vi "Handle.vi"(11 "Hello World Queue in":refnum<class "Hello World Queue.lvclass">) -> (2 "Destroy?":bool, 3 "Hello World Queue out":refnum<class "Hello World Queue.lvclass">)   [LabVIEW 2021, in "Hello World Queue.lvlib" / "Hello World Queue.lvclass"]
uses:
  Hello World Queue.lvclass
  Hello World Queue.lvclass/Hello World Queue.ctl
  jettl/Actor/Queue Actor/Queue Actor.lvclass
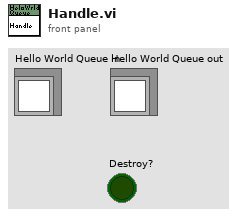
[diagram p1: front panel]
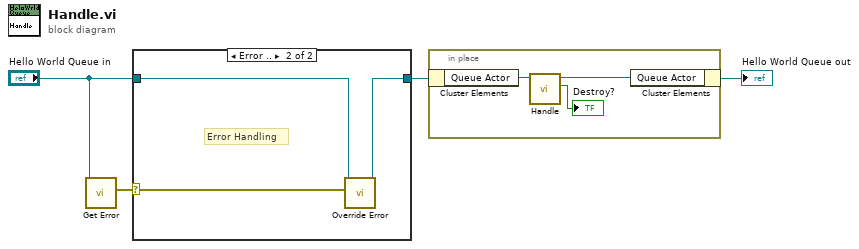
[diagram p0: block diagram]
diagram:
  n1 = call-dynamic "Get Error.vi"("Hello World Queue in"="Hello World Queue in") -> ("Error"=w4:errorcluster)  [unwired: 10 in]
  n2 = case shown="Error .." w4 {
    selector: w4 -> [_ w6]
    tunnel: "Hello World Queue in" -> [w5 w8]
    tunnel: [w5 w7] -> w2
    frame No Error {
    }
    frame Error {
      # "Error Handling"
      n3 = call-dynamic "Override Error.vi"("Error"=w6, "Hello World Queue in"=w8) -> ("Hello World Queue out"=w7:refnum<class "Hello World Queue.lvclass">)  [unwired: 9 in]
    }
  }
  n4 = in-place {
    n5 = in-place-cluster #1(w2) -> ("Queue Actor"=w11:refnum<class "Queue Actor.lvclass">)
    n6 = call-dynamic "Handle.vi"("Actor in"=w11) -> ("Destroy?"=→"Destroy?":bool, "Actor out"=w10:refnum<class "Queue Actor.lvclass">)  [unwired: 9 in]
    n7 = in-place-cluster #1("Queue Actor"=w10) -> (→"Hello World Queue out":refnum<class "Hello World Queue.lvclass">)
  }
